vi "MT Generate CPM System Parameters.vi"   [LabVIEW 2020, in "niDMT.lvlib"]
doc: "This VI calculates parameters for use with either the MT Modulate CPM VI or the MT Demodulate CPM VI."
uses:
  <vilib>/addons/Modulation/niDMT.lvlib
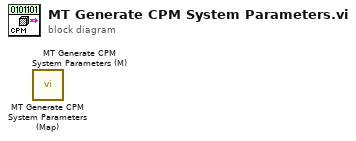
[diagram p0: block diagram]
diagram:
  n1 = call <vilib>:"MT Generate CPM System Parameters (Map).vi"() -> ()  [unwired: 14 in, 2 out]
  n2 = call <vilib>:"MT Generate CPM System Parameters (M).vi"() -> ()  [unwired: 13 in, 3 out]
